vi "Configure Import Waveform.vi"(2 "data format":T1=enum."Binary", 4 "Set Waveform Name":string, 5 "Specify the  Waveform Type":u16(ring) items=["Analog", "Digitals"], 6 "Digital Waveform In":digitalwaveform(waveform), 7 "Select  File Name (Absolute Path) to Import from AWG's Files System":path, 8 "error in (no error)":errorcluster, 9 "wave in":dbl[](array[numeric]), 10 "Import Waveform":bool, 11 "VISA resource name":refnum<visa-resource-name>) -> (0 "error out":errorcluster, 3 "VISA resource name out":refnum<visa-resource-name>)   [LabVIEW 2020, in "Active Technologies AWG3000.lvlib"]
uses:
  Active Technologies AWG3000.lvlib
  711169be-9fd4-4b71-8deb-500df821156a.vi
  <vilib>/Waveform/DWDTOps.llb/DWDT Digital to Binary U32.vi
  <vilib>/Comparison/Equal/Equal Functor/Equal Functor.lvclass
panel:
  out "temp file name":string
  out "data string":string
  out "Default Import/Export Folder for Drive C":path
  # "After setting these parameters and launching the VI, if errors do not appear in the Error Out Indicator, a new waveform with a name specified in the box on the side  will be present in the Waveforms List and it will be possible to insert it in the sequencer entries."
  # "Import from File"
  # "Run this Vi to know the default folder for Drive C from which to import the file. Remember that for Drive C  is allowed import a file only from the default folder or its subdirectories."
  # "Choose .txt or .trc file specifing its absolute path. Remember the note above if the file to be imported is located in Drive C."
  # "Import with a Data Transfer (Analog Waveform)"
  # "Import with a Data Transfer (Digital Waveform)"
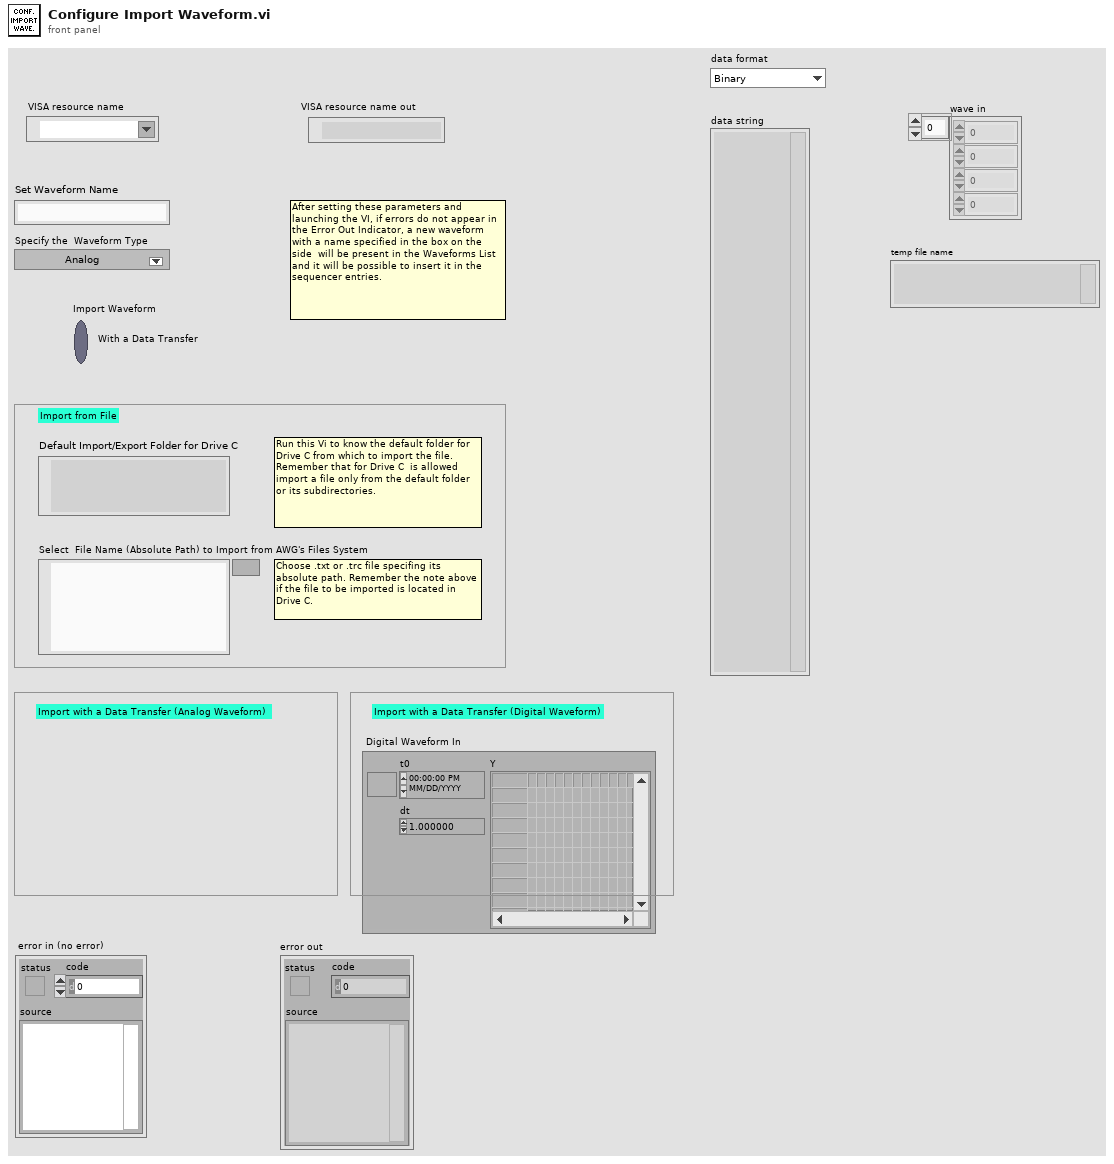
[diagram p1: front panel]
types:
  T1 = typedef "Active Technologies AWG3000.lvlib/T3AWG Wave Format" = enum16{"Text", "Binary"}
  T2 = enum16{"big-endian, network order", "native, host order", "little-endian"}
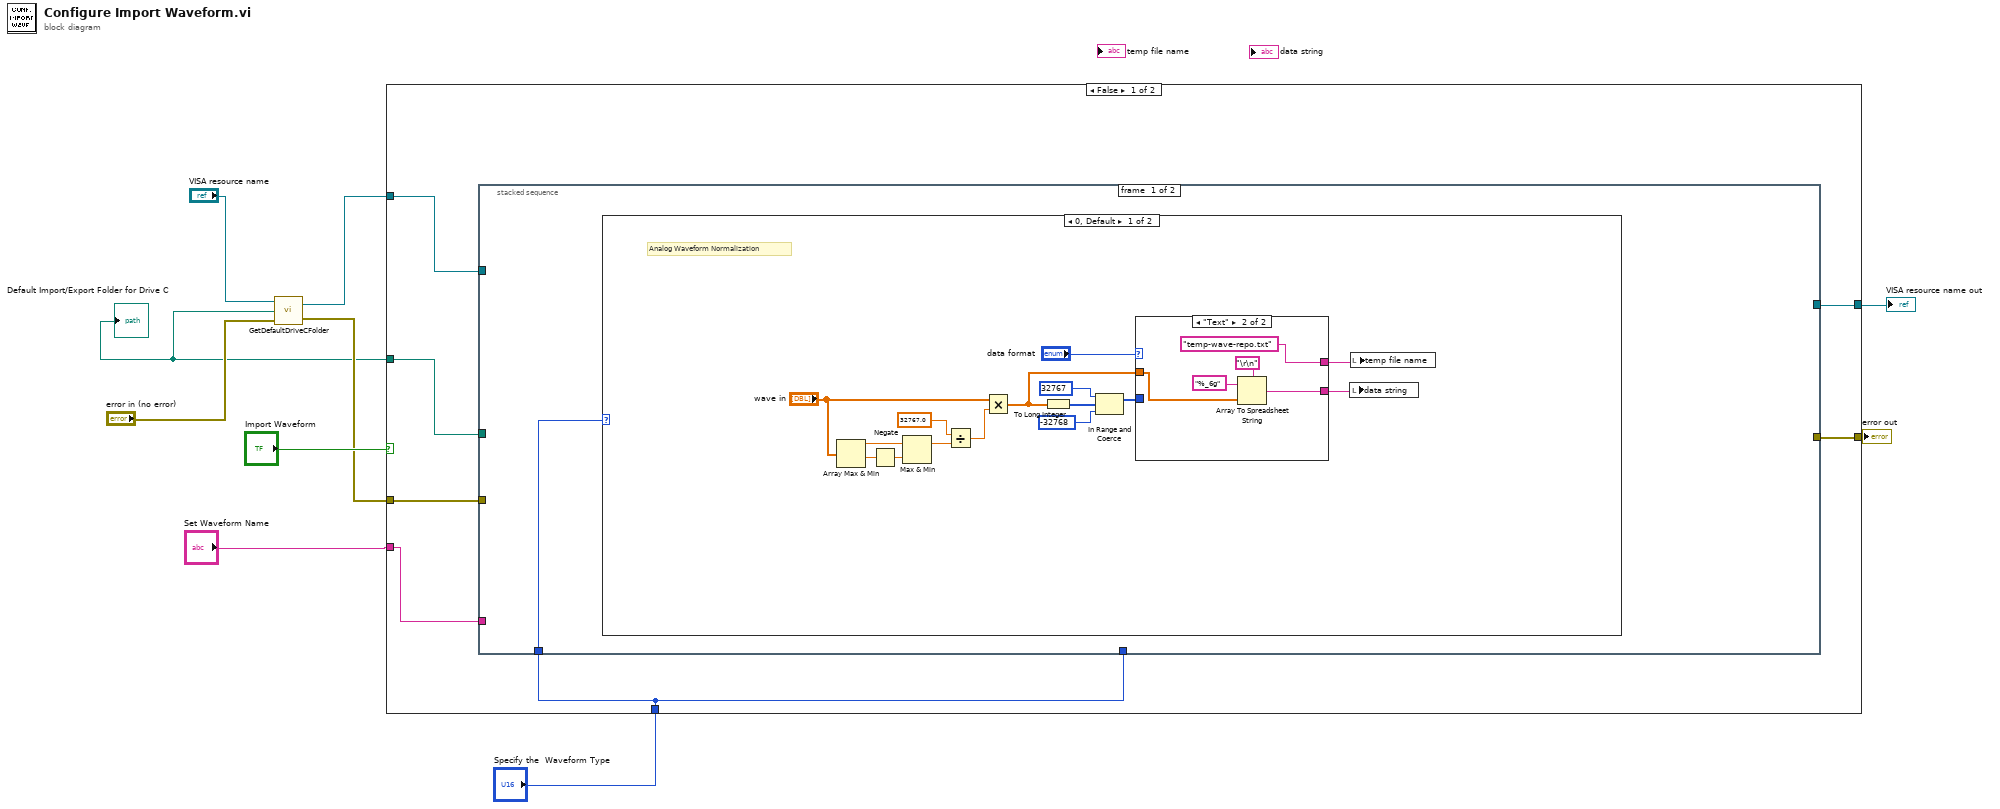
[diagram p0: block diagram]
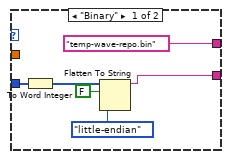
[diagram p2: hidden frame]
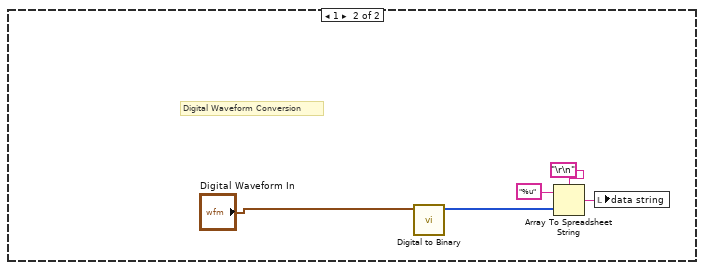
[diagram p3: hidden frame]
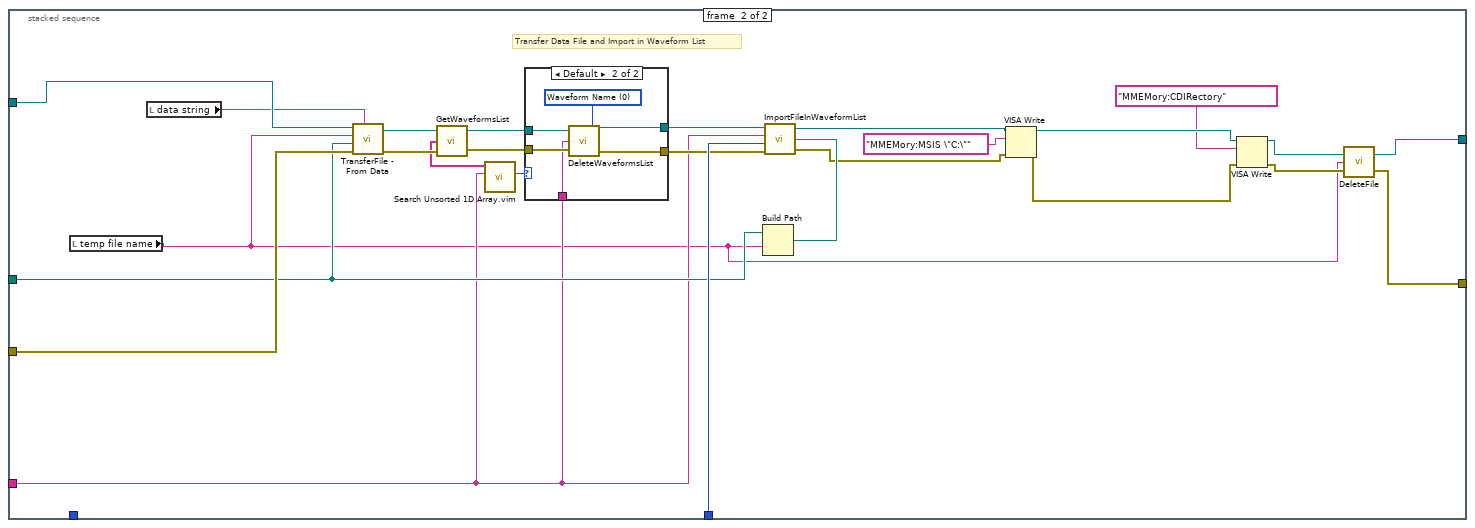
[diagram p4: hidden frame]
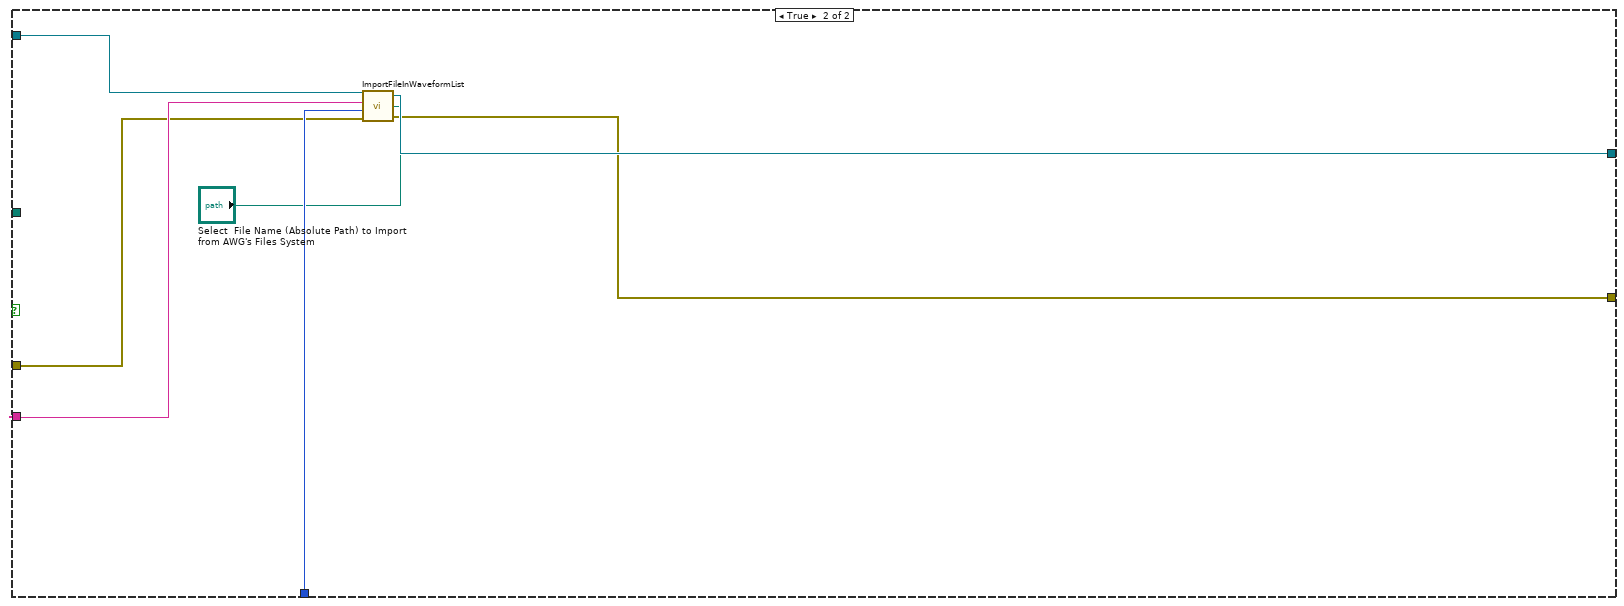
[diagram p6: hidden frame]
diagram:
  n1 = call "GetDefaultDriveCFolder.vi"("error in (no error)"="error in (no error)", "VISA resource name"="VISA resource name") -> ("error out"=w3:errorcluster, "VISA resource name out"=w4:refnum<visa-resource-name>, "Default Import/Export Folder for Drive C"=w2:path)
  "Default Import/Export Folder for Drive C" <- w2
  n2 = case shown="False" "Import Waveform" {
    tunnel: w3 -> [w16 w85]
    tunnel: w4 -> [w17 w84]
    tunnel: [w13 w90] -> w9
    tunnel: [w14 w89] -> w8
    tunnel: "Specify the  Waveform Type" -> [w11 w88]
    tunnel: "Set Waveform Name" -> [w12 w86]
    tunnel: w2 -> [w15 _]
    frame False {
      n3 = stacked-sequence {
        tunnel: w17 -> [_ w62]
        tunnel: w16 -> [_ w63]
        tunnel: w15 -> [_ w61]
        tunnel: w12 -> [_ w52]
        tunnel: w11 -> [_ w75]
        tunnel: [_ w73] -> w13
        tunnel: [_ w72] -> w14
        tunnel: w11 -> [w18 _]
        frame #0 {
          n4 = case shown="0, Default" w18 {
            frame 0, Default {
              # "Analog Waveform Normalization"
              n5 = Array Max & Min(array="wave in") -> (max value=w23:dbl, min value=w25:dbl)  [unwired: 2 out]
              n6 = Negate(x=w25) -> (-x=w24:dbl)
              n7 = Max & Min(x=w23, y=w24) -> (max(x,y)=w20:dbl)  [unwired: 1 out]
              n8 = Divide(x=32767.0, y=w20) -> (x/y=w22:dbl)
              n9 = Multiply(x="wave in", y=w22) -> (x*y=w19:dbl[])
              n10 = To Long Integer(number=w19) -> (32bit integer=w33:i32[])
              n11 = In Range and Coerce(upper limit=32767, x=w33, lower limit=-32768) -> (coerced(x)=w32:i32[])  [unwired: 1 out]
              n12 = case shown="\"Text\"" "data format" {
                tunnel: [w35 w42] -> w28
                tunnel: w32 -> [w39 _]
                tunnel: ["temp-wave-repo.bin" ("temp file name") "temp-wave-repo.txt" ("temp file name")] -> w27
                tunnel: w19 -> [_ w40]
                frame "Binary" {
                  n13 = To Word Integer(number=w39) -> (16bit integer=w38:i16[])
                  n14 = Flatten To String(anything=w38, prepend array or string size? (T)=FALSE, byte order (0:big-endian, network order)=T2."little-endian") -> (data string=w35:string)  [unwired: 1 in, 2 out]
                }
                frame "Text" {
                  n15 = Array To Spreadsheet String(delimiter (Tab)="\r\n", array=w40, 3:"%_6g" ("format (%.3f)")) -> (spreadsheet string=w42:string)
                }
              }
              n16 = local write "data string"(w28) -> ()
              n17 = local write "temp file name"(w27) -> ()
            }
            frame 1 {
              # "Digital Waveform Conversion"
              n18 = call-poly <vilib>:"Digital to Binary.vi"("digital waveform"="Digital Waveform In") -> ("binary array"=w46:u32[])  [unwired: 9 in, 1 out]
              n19 = Array To Spreadsheet String(delimiter (Tab)="\r\n", array=w46, 3:"%u" ("format (%.3f)")) -> (spreadsheet string=w48:string)
              n20 = local write "data string"(w48) -> ()
            }
          }
        }
        frame #1 {
          # "Transfer Data File and Import in Waveform List"
          n21 = local read "temp file name"() -> (w50:string)
          n22 = local read "data string"() -> (w60:string)
          n23 = call "TransferFile - From Data.vi"("data in"=w60, "error in (no error)"=w63, "Choose the Destination File Folder (Absolute Path) for AWG's files system"=w61, "Set File Name (with Extension)"=w50, "VISA resource name"=w62) -> ("error out"=w57:errorcluster, "VISA resource name out"=w56:refnum<visa-resource-name>)  [unwired: 5 in]
          n24 = call "GetWaveformsList.vi"("error in (no error)"=w57, "VISA resource name"=w56) -> ("error out"=w55:errorcluster, "VISA resource name out"=w54:refnum<visa-resource-name>, "Waveforms List"=w53:string[])
          n25 = call "Search Unsorted 1D Array.vim"("element"=w52, "unsorted 1D array"=w53) -> ("index of element"=w51:i32)  [unwired: 9 in]
          n26 = case shown="Default" w51 {
            tunnel: [w77 w82] -> w59
            tunnel: [w76 w81] -> w58
            tunnel: w55 -> [w77 w80]
            tunnel: w54 -> [w76 w79]
            tunnel: w52 -> [_ w78]
            frame -1 {
            }
            frame Default {
              w83 = u16 0 items=["Waveform Name", "All (Only Imported Waveforms)"] ("Delete Waveform Options")
              n27 = call "DeleteWaveformsList.vi"("Delete Waveform Options"=w83, "error in (no error)"=w80, "Delete Waveform from Waveform List (Name)"=w78, "VISA resource name"=w79) -> ("error out"=w82:errorcluster, "VISA resource name out"=w81:refnum<visa-resource-name>)
            }
          }
          n28 = Build Path(base path=w61, name or relative path=w50) -> (appended path=w74:path)
          n29 = call "ImportFileInWaveformList.vi"("Select  File Name (Absolute Path) to Import  from AWG's Files System"=w74, "error in (no error)"=w59, "Specify the  Waveform Type"=w75, "Set the Waveform Name"=w52, "VISA resource name"=w58) -> ("error out"=w70:errorcluster, "VISA resource name out"=w69:refnum<visa-resource-name>)
          n30 = VISA Write(VISA resource name=w69, write buffer="MMEMory:MSIS \"C:\"", error in (no error)=w70) -> (VISA resource name out=w68:refnum<visa-resource-name>, error out=w67:errorcluster)  [unwired: 1 out]
          n31 = VISA Write(VISA resource name=w68, write buffer="MMEMory:CDIRectory", error in (no error)=w67) -> (VISA resource name out=w66:refnum<visa-resource-name>, error out=w65:errorcluster)  [unwired: 1 out]
          n32 = call "DeleteFile.vi"("error in (no error)"=w65, "File Name (with Extension)"=w50, "VISA resource name"=w66) -> ("error out"=w72:errorcluster, "VISA resource name out"=w73:refnum<visa-resource-name>)
        }
      }
    }
    frame True {
      n33 = call "ImportFileInWaveformList.vi"("Select  File Name (Absolute Path) to Import  from AWG's Files System"="Select  File Name (Absolute Path) to Import from AWG's Files System", "error in (no error)"=w85, "Specify the  Waveform Type"=w88, "Set the Waveform Name"=w86, "VISA resource name"=w84) -> ("error out"=w89:errorcluster, "VISA resource name out"=w90:refnum<visa-resource-name>)
    }
  }
  "VISA resource name out" <- w9
  "error out" <- w8
